vi "Load Images.vi"(8 "error in (no error)":errorcluster, 11 "images Folder":path) -> (0 "error out":errorcluster)   [LabVIEW 2020, in "TSnax UI.lvlib" / "TSnax UI Manager.lvclass"]
uses:
  TSnax UI Manager.lvclass
  Image.ctl
  TSnax UI Manager.lvclass/TSnax UI Manager.ctl
  TSnax UI.lvlib
panel:
  out "Pictures":picture[](array[picture])
  out "Image Names":string[](array[string])
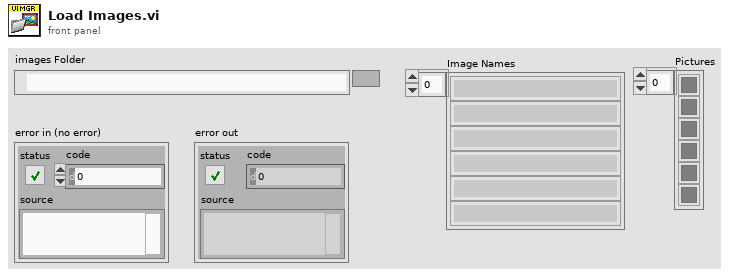
[diagram p1: front panel]
types:
  T1 = typedef "TSnax UI.lvlib/Image.ctl" = enum16{"YellowArrow", "GreenArrow"}
  T2 = typedef "imagedata.ctl" = cluster{"image type":i32, "image depth":i32, "image":u8[], "mask":u8[], "colors":u32[], "Rectangle":cluster{"left":i16, "top":i16, "right":i16, "bottom":i16}}
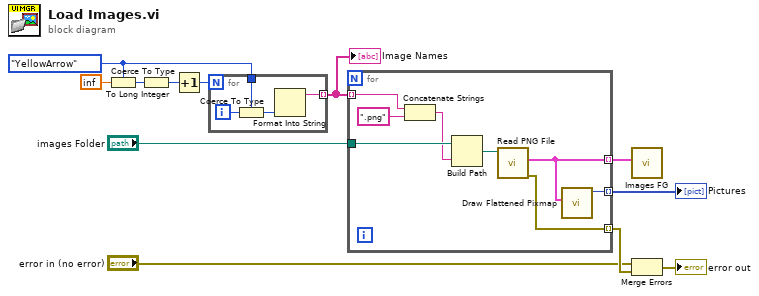
[diagram p0: block diagram]
diagram:
  w9 = Image."YellowArrow" ("Image")
  n1 = Coerce To Type(0:inf, 1:w9) -> (2:w11:T1)
  n2 = To Long Integer(number=w11) -> (32bit integer=w10:i32)
  n3 = Increment(x=w10) -> (x+1=w8:i32)
  n4 = for {
    N: w8 -> [_]
    tunnel: w9 -> [w15]
    tunnel: [w13] -> w7 mode=indexing
    i -> [w16]
    n5 = Coerce To Type(0:w16, 1:w15) -> (2:w14:T1)
    n6 = Format Into String(w14) -> (resulting string=w13:string)  [unwired: 3 in, 1 out]
  }
  "Image Names" <- w7
  n7 = for {
    tunnel: w7 -> [w24] mode=indexing
    tunnel: "images Folder" -> [w22]
    tunnel: [w19] -> w1 mode=indexing
    tunnel: [w18] -> w5 mode=indexing
    tunnel: [w17] -> w4 mode=indexing
    n8 = Concatenate Strings(w24, ".png" ("string")) -> (w21:string)
    n9 = Build Path(base path=w22, name or relative path=w21) -> (appended path=w20:path)
    n10 = call <vilib>:"Read PNG File.vi"("path to PNG file"=w20) -> ("error out"=w17:errorcluster, "image data"=w19:T2)  [unwired: 8 in, 1 out]
    n11 = call <vilib>:"Draw Flattened Pixmap.vi"("image data"=w19) -> ("new picture"=w18:picture)  [unwired: 8 in]
  }
  "Pictures" <- w5
  n12 = call "Images FG.vi"("All Images In"=w1) -> ()  [unwired: 10 in, 1 out]
  n13 = Merge Errors("error in (no error)", w4) -> (→"error out":errorcluster)
